vi "Configure Resistance Measurement Type.vi"(8 "error in (no error)":errorcluster, 10 "Measurement Type (0: Normal)":i32(ring) items=["Normal", "Resistivity"], 11 "VISA resource name":refnum<visa-resource-name>) -> (0 "error out":errorcluster, 3 "VISA resource name out":refnum<visa-resource-name>)   [LabVIEW 2020, in "Keithley 6517.lvlib"]
doc: "Configures resistance measurement type.\n\n<B>Note:</B>\nThis VI is <B>NOT</B> compatible with model <B>6514</B>."
uses:
  <instrlib>/Keithley 6517/Keithley 6517.lvlib
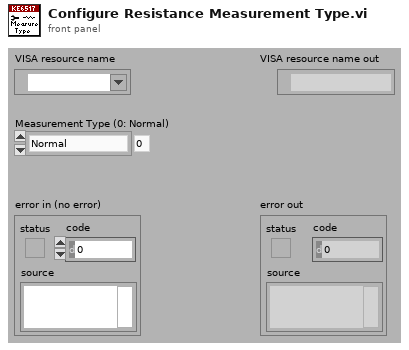
[diagram p1: front panel]
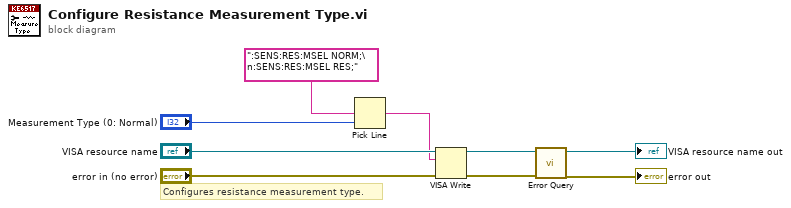
[diagram p0: block diagram]
diagram:
  # "Configures resistance measurement type."
  n1 = Pick Line(multi-line string=":SENS:RES:MSEL NORM;\n:SENS:RES:MSEL RES;", line index="Measurement Type (0: Normal)") -> (output string=w2:string)  [unwired: 1 in]
  n2 = VISA Write(VISA resource name="VISA resource name", write buffer=w2, error in (no error)="error in (no error)") -> (VISA resource name out=w7:refnum<visa-resource-name>, error out=w6:errorcluster)  [unwired: 1 out]
  n3 = call <instrlib>:"Error Query.vi"("error in (no error)"=w6, "VISA resource name"=w7) -> ("error out"=→"error out":errorcluster, "VISA resource name out"=→"VISA resource name out":refnum<visa-resource-name>)  [unwired: 6 in, 2 out]
